vi "Easy_Test2.vi"(8 "Stop":bool, 10 "Boolean In":bool) -> (2 "Boolean Out":bool)   [LabVIEW 2014]
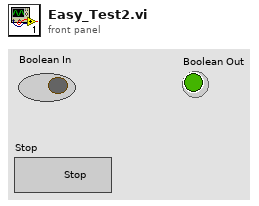
[diagram p1: front panel]
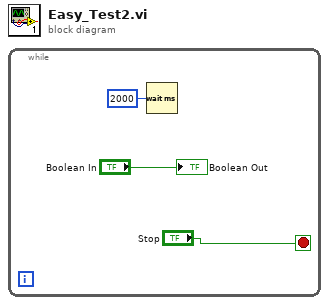
[diagram p0: block diagram]
diagram:
  n1 = while {
    stop <- "Stop" stop-if-true
    n2 = Wait (ms)(milliseconds to wait=u32 2000) -> ()  [unwired: 1 out]
    "Boolean Out" <- "Boolean In"
  }
